vi "sensor de temperatura humedad dth11.vi"() -> ()   [LabVIEW 2016]
uses:
  <vilib>/LabVIEW Interface for Arduino/Type Defs/Board Type.ctl
  <vilib>/LabVIEW Interface for Arduino/Type Defs/Connection Type.ctl
  <vilib>/LabVIEW Interface for Arduino/LabVIEW Interface for Arduino.lvlib
  Read Data V14/DHTXX.lvlib
panel:
  in  "?":bool
  out "Lectura":bool
  out "Humedad(%)":dbl(slide) scale=0.0..100.0
  out "Temperatura(C)":dbl(slide) scale=0.0..50.0
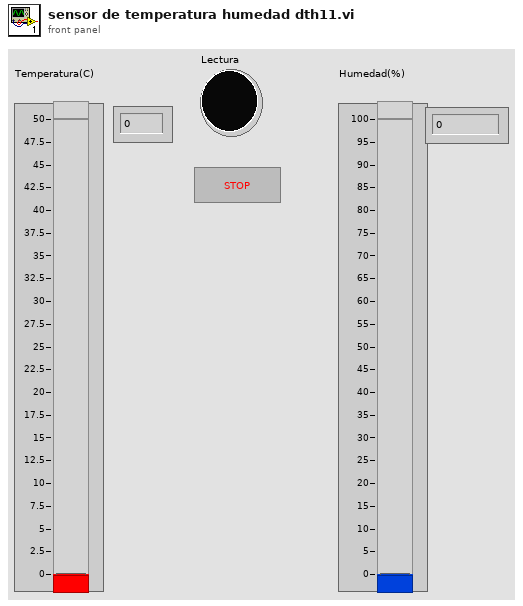
[diagram p1: front panel]
types:
  T1 = typedef "LabVIEW Interface for Arduino.lvlib/Connection Type.ctl" = enum8{"USB / Serial", "XBEE", "BlueSmirf (Bluetooth)"}
  T2 = typedef "LabVIEW Interface for Arduino.lvlib/Board Type.ctl" = enum16{"Uno", "Dimuelanove w/Atmega 328", "Mega 2560"}
  T3 = typedef "LabVIEW Interface for Arduino.lvlib/Arduino Resource.ctl" = cluster{"VISA resource":refnum<visa-resource-name>, "Board Type":T2, "Connection Type":enum8{"USB / Serial"}, "Bytes Per Packet (15)":u8}
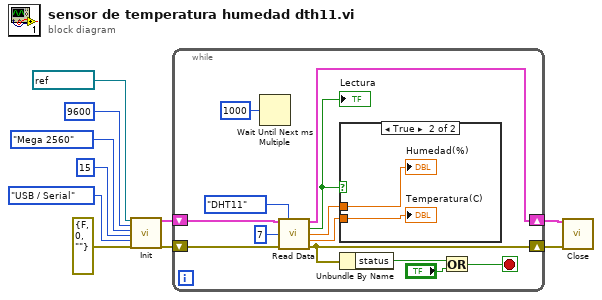
[diagram p0: block diagram]
diagram:
  n1 = call <vilib>:"Init.vi"("VISA resource"=refnum<visa-resource-name> "COM8", "Baud Rate (115200)"=u32 9600, "Board Type (Uno)"=Board_Type."Mega 2560", "Bytes Per Packet (15)"=u32 15, "Connection Type (USB/Serial)"=Connection_Type."USB / Serial", "error in"=errorcluster {"status"=FALSE, "code"=0, "source"=""}) -> ("Arduino Resource"=w4:T3, "error out"=w3:errorcluster)  [unwired: 12 in]
  n2 = while {
    shift-right: [w18] -> w1
    shift-left: w4 -> [w23]
    shift-right: [w12] -> w2
    shift-left: w3 -> [w22]
    stop <- w15 stop-if-true
    n3 = Wait Until Next ms Multiple(millisecond multiple=u32 1000) -> ()  [unwired: 1 out]
    n4 = call "Read Data.vi"("Arduino Resource"=w23, "Sensor Type"=enum16{"DHT11", "DHT21", "DHT22"}."DHT11", "Pin"=u8 7, "error in (no error)"=w22) -> ("Arduino Resource"=w18:T3, "Successful?"=w19:bool, "Relative Humidity"=w17:dbl, "Temperature (°C)"=w16:dbl, "error out"=w12:errorcluster)  [unwired: 7 in]
    "Lectura" <- w19
    n5 = case shown="True" w19 {
      tunnel: w17 -> [_ w25]
      tunnel: w16 -> [_ w24]
      frame False {
      }
      frame True {
        "Temperatura(C)" <- w24
        "Humedad(%)" <- w25
      }
    }
    n6 = Unbundle By Name(w12) -> ("status"=w13:bool)
    n7 = Or(x=w13, y="?") -> (x .or. y?=w15:bool)
  }
  n8 = call <vilib>:"Close.vi"("Arduino Resource"=w1, "error in"=w2) -> ()  [unwired: 13 in, 1 out]
